vi "Add VIs from Target.vi"(9 "VI Queue":refnum<queue>, 10 "Target":refnum<vi>, 11 "Search":refnum<class "Search.lvclass">) -> ()   [LabVIEW 2020, in "Better Search.lvlib" / "Search.lvclass"]
uses:
  Search.lvclass
  Search.lvclass/Search.ctl
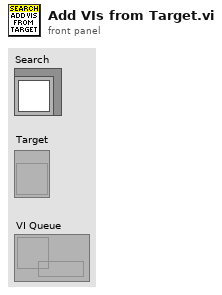
[diagram p1: front panel]
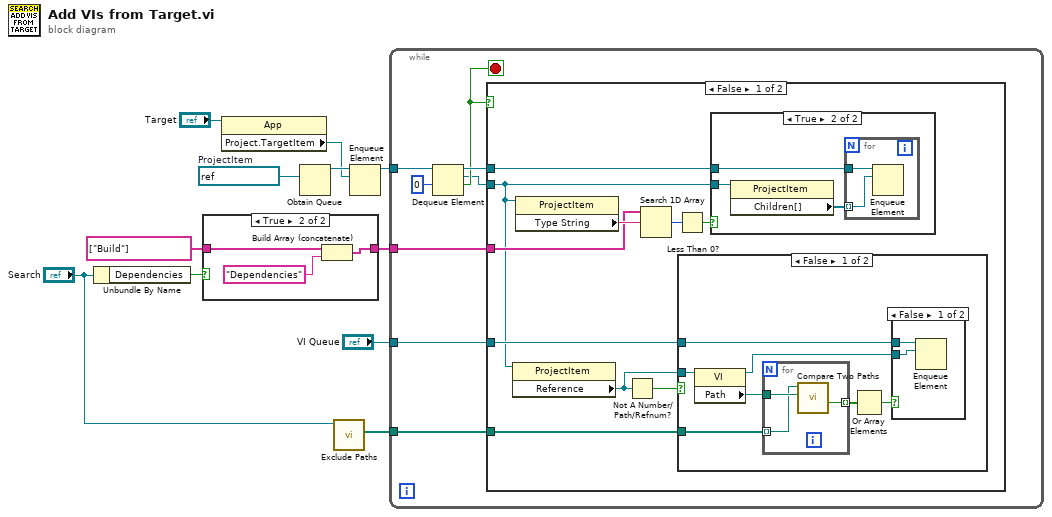
[diagram p0: block diagram]
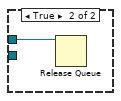
[diagram p6: hidden frame]
diagram:
  w2 = refnum<vi> refnum  # ProjectItem
  n1 = Unbundle By Name("Search") -> ("Dependencies"=w6:bool)
  n2 = case shown="True" w6 {
    tunnel: string[] ["Build"] -> [w12 w15]
    tunnel: [w12 w13] -> w5
    frame False {
    }
    frame True {
      n3 = Build Array (concatenate)(w15, "Dependencies") -> (w13:string[])
    }
  }
  n4 = property class="App"(reference="Target") -> ("Project.TargetItem"=w1:refnum<vi>)  [unwired: 1 in, 2 out]
  n5 = Obtain Queue(element data type=w2) -> (queue out=w10:refnum<queue>)  [unwired: 4 in, 2 out]
  n6 = call "Exclude Paths.vi"("Search in"="Search") -> ("Exclude Paths"=w4:path[])  [unwired: 8 in, 2 out]
  n7 = Enqueue Element(queue=w10, element=w1) -> (queue out=w9:refnum<queue>)  [unwired: 2 in, 2 out]
  n8 = while {
    tunnel: "VI Queue" -> [w18]
    tunnel: w9 -> [w23]
    tunnel: w5 -> [w17]
    tunnel: w4 -> [w16]
    stop <- w20 stop-if-true
    n9 = Dequeue Element(queue=w23, timeout in ms (-1)=0) -> (queue out=w21:refnum<queue>, element=w19:refnum<vi>, timed out?=w20:bool)  [unwired: 1 in, 1 out]
    n10 = case shown="False" w20 {
      tunnel: w21 -> [w33 w51]
      tunnel: w19 -> [w27 _]
      tunnel: w18 -> [w32 _]
      tunnel: w17 -> [w28 _]
      tunnel: w16 -> [w24 _]
      frame False {
        n11 = property class="ProjectItem"(reference=w27) -> ("Reference"=w31:refnum<vi>)  [unwired: 1 in, 2 out]
        n12 = property class="ProjectItem"(reference=w27) -> ("Type String"=w29:string)  [unwired: 1 in, 2 out]
        n13 = Not A Number/Path/Refnum?(number/path/refnum=w31) -> (NaN/Path/Refnum?=w30:bool)
        n14 = Search 1D Array(1D array=w28, element=w29) -> (index of element=w26:i32)  [unwired: 1 in]
        n15 = Less Than 0?(x=w26) -> (x < 0?=w25:bool)
        n16 = case shown="False" w30 {
          tunnel: w32 -> [w45 _]
          tunnel: w31 -> [w44 _]
          tunnel: w24 -> [w42 _]
          frame False {
            n17 = property class="VI"(reference=w44) -> (reference out=w39:refnum<vi>, "Path"=w43:path)  [unwired: 1 in, 1 out]
            n18 = for {
              tunnel: w43 -> [w50]
              tunnel: w42 -> [w49] mode=indexing
              tunnel: [w48] -> w41 mode=indexing
              n19 = call <vilib>:"Compare Two Paths.vi"("Path 2"=w50, "Path 1"=w49) -> ("Path 2 Relative to Path 1?"=w48:bool)  [unwired: 6 in, 3 out]
            }
            n20 = Or Array Elements(Boolean array=w41) -> (logical OR=w40:bool)
            n21 = case shown="False" w40 {
              tunnel: w45 -> [w47 _]
              tunnel: w39 -> [w46 _]
              frame False {
                n22 = Enqueue Element(queue=w47, element=w46) -> ()  [unwired: 2 in, 3 out]
              }
              frame True {
              }
            }
          }
          frame True {
          }
        }
        n23 = case shown="True" w25 {
          tunnel: w33 -> [_ w36]
          tunnel: w27 -> [_ w34]
          frame False {
          }
          frame True {
            n24 = property class="ProjectItem"(reference=w34) -> ("Children[]"=w35:refnum<vi>[])  [unwired: 1 in, 2 out]
            n25 = for {
              tunnel: w35 -> [w37] mode=indexing
              tunnel: w36 -> [w38]
              n26 = Enqueue Element(queue=w38, element=w37) -> ()  [unwired: 2 in, 3 out]
            }
          }
        }
      }
      frame True {
        n27 = Release Queue(queue=w51) -> ()  [unwired: 2 in, 3 out]
      }
    }
  }
